vi "ADC Get Capabilities.vi"(7 "Initialize HW? (False)":bool, 8 "error in":errorcluster, 10 "parameters":T1, 11 "adc session in":T5={"niScope"={"channel cfg"=[], "sessions"=[], "multi cards"=FALSE, "channels"=0, "type"=enum."n/a", "memory [B/chn]"=0, "ext. clock [Hz]"=0.0, "samples count"=0, "use streaming"=FALSE, "proc setup"={"packet size [smpl]"=0, "current timeout [s]"=0.0, "blk2blk timeout [s]"=0.0, "event time"=timestamp(0 s since 1904-01-01), "temp sampl T [s]"=0.0, "data queue"=refnum, "stop notifier"=refnum, "proc ref"=refnum}, "sample width [B]"=0, "ranges [V]"=[], "trigger setup"={"coupling"=1, "level [V]"=0.0, "slope"=0, "mode"=enum."Immediate", "pre-trigger [%]"=0.0}, "fs [Hz]"=0.0, "bitres [bit]"=0, "clock source"=enum."VAL_NO_SOURCE"}, "3458A"={"channels"=[], "sync unit"={"VISA"="", "type"=enum."Picotest U6200A"}, "awg unit"={"type"=enum."Agilent 331xxA to 332xxA", "VISA"="", "enable 10MHz ref"=FALSE, "cmi ckd2"={"VISA"="", "clock source"=enum."Auto", "manual ref clk"=FALSE, "ref clock [Hz]"=0.0, "div mode"=enum."Set divisor directly"}, "cmi sync v3"={"VISA"="", "baud rate [bd/s]"=115200, "source"=enum."Auto", "hv range"=enum."1kV", "fsrc is fixed"=FALSE, "fsrc [Hz]"=10000000.0, "freq integ [s]"=1.0, "freq filter"=5, "trig level"=enum."TTL 5V", "chn1 mode"=enum."Source divider", "chn1 level"=enum."Positive 5V", "chn2 mode"=enum."Source divider", "chn2 level"=enum."Positive 5V", "chn2 div"=1, "chn3 mode"=enum."Chn 1 Active", "chn3 level"=enum."Positive 5V", "chn1 div entry"=enum."Calculate nearest divisor from measured fx", "chn1 dev limit [%]"=1.0, "chn1 check dev"=FALSE}, "trigger"={"source"=enum."Immediate", "slope"=enum."POS", "coupling"=enum."DC", "level [V]"=0.0, "hysteresis [V]"=0.0, "pre-trigger [%]"=0.0}, "HMF2500 cfg"={"Baud Rate"=9600, "Parity"=0, "Data Bits"=8, "Flow Control"=4}}, "sync mode"=enum."MASTER-SLAVE, MASTER clocked by TIMER", "streaming mode"=FALSE, "idn mode"=enum."Auto", "sampling mode"=enum."DCV", "sample memory [B]"=0, "proc setup"={"channel id"=0, "packet size [smpl]"=0, "current timeout [s]"=0.0, "blk2blk timeout [s]"=0.0, "event time"=timestamp(0 s since 1904-01-01), "stop notifier"=refnum, "data queues"=[], "proc refs"=[], "bus semaphore"=refnum}, "sample size [B]"=0, "sample count"=0, "aux data"={"channel id"=0, "valid?"=[], "gain [V]"=[], "timestamp [s]"=[], "Ts [s]"=0.0, "abs timestamp"=timestamp(0 s since 1904-01-01), "t [deg C]"=[], "multiplex timestamp [s]"=-1.0, "only multiplex?"=FALSE, "multiplex smpl offset"=0, "overflow?"=FALSE}, "ranges [V]"=[], "aperture [s]"=0.0, "LEVEL trigger"={"edge"=enum."POS", "level [V]"=0.0, "coupling"=enum."DC"}, "trigger mode"=enum."AUTO", "measure temp.?"=FALSE, "disp mesages"=[], "shared bus?"=FALSE, "disable display?"=FALSE, "aper mode"=enum."Manual", "aper rules"=[], "multiplex"={"cycles"=0, "delay [s]"=0.0, "enabled"=FALSE, "overhead [s]"=1.0, "tot smpls"=0, "sub-rec"=0, "overhead [%]"=0.0, "emulated"=FALSE}, "F8588 lpf"=enum."Off", "F8588 pll"=enum."Off", "F8588 couple"=enum."DC, auto", "fs"={"freq mode"=enum."fs or Ts", "fs [Hz]"=0.0, "fref [Hz]"=0.0, "mul"=0.0, "div"=0.0}, "fs mode"=enum."fs or Ts"}, "dsdll"={"dsdll"={"dsdll path"=path "", "dsdll handle"=[], "output devices"=[], "capture devices"=[]}, "channels"=0, "device id"=0, "channel idns"=[], "proc setup"={"packet size [smpl]"=0, "current timeout [s]"=0.0, "blk2blk timeout [s]"=0.0, "event time"=timestamp(0 s since 1904-01-01), "data queue"=refnum, "stop notifier"=refnum, "proc ref"=refnum}, "samples count"=0, "fs [Hz]"=0.0}, "type"=enum."niScope", "channel idn str"=[], "aux instr idn str"=[], "modified?"=FALSE, "simadc"={"channels"=[], "range [V]"=0.0, "Ts step [s]"=0.0, "time [s]"=0.0, "fs [Hz]"=0.0, "count"=0, "smpl offset"=0, "set count"=0, "bit res"=0}, "force rst?"=FALSE, "exit mode"=enum."Immediate reset", "exit dly"=0.0, "exit tmr"=timestamp(0 s since 1904-01-01), "busy?"=FALSE, "accessed?"=FALSE, "multiplex"={"Type"=enum."Dummy", "gen com ssn"={"visa"="", "primary"=enum."None", "secondary"=enum."None", "channels"=[]}, "delay before [s]"=0.0, "delay post [s]"=0.0, "sequence"=[], "enabled"=FALSE, "ref timestamp [s]"=0.0, "idn string"="", "dev niScope"="", "niScope idx"=0, "QPMX ssn"={"visa"="", "switch mode"=enum."Switched by TWM", "sequence"=[], "timing delays"=[], "polarity"=enum."Positive", "ss delay (s)"=2.0, "internal timer (s)"=1.0, "Last loaded sequence file"=path "", "startup delay (s)"=2.0}, "VISA mux ssn"={"VISA"="", "paths"=[], "idn command"="", "serial cfg"={"Baud rate"=9600, "Data bits"=8, "Parity"=0, "Stop bits"=10, "Flow control"=0, "End Mode Read"=enum."None", "End Mode Write"=enum."None", "Term character"=0, "Term enable"=FALSE}}}, "keysight dso"={"VISA"="", "channels"=[], "bw limit [Hz]"=0.0, "resolution"=enum."Basic", "trig noise reject"=enum."Normal", "N"=0, "trigger config"={"trigger source"=enum."Immediate", "trigger slope"=enum."Negative", "level [V]"=0.0, "hysteresis [V]"=0.001, "pre-trig [%]"=50}, "fs [Hz]"=0.0, "timeout stop"=timestamp(0 s since 1904-01-01), "waiting for opc"=FALSE, "fetch offset [smpl]"=0, "abs timestamp"=timestamp(0 s since 1904-01-01), "ranges [V]"=[], "decimation"=1.0, "ext ref"=FALSE, "emulate aperture"=FALSE, "model"=enum."DSO91304"}, "cdaq"={"mclk [Hz]"=12800000.0, "ADC task"="", "mclk reference"="", "fs [Hz]"=50000.0, "queue adc cmd"=refnum, "queue adc data"=refnum, "adc proc ref"=refnum, "channels"=[], "last channels"=[], "timeout"=timestamp(0 s since 1904-01-01), "N"=1000, "mclk mode"=enum."Free running", "ext mclk source"=""}, "ignore overload"=FALSE, "ADS127L21"={"VISA"="", "chn list"=[], "record size"=0, "phys. channels"=0, "adc fifo size"=0, "channels"=[], "ext refclk?"=FALSE, "fs [Hz]"=0.0, "ext refclk [Hz]"=0.0, "meas refclk [Hz]"=0.0, "EXTOUT mode"=enum."ADCCLK", "EXTOUT polarity"=enum."NORM", "EXTOUT divisor"=0}} {"ADS127L21"."channels"."Channel" min=1 max=8 step=1; "cdaq"."last channels"."Channel id" min=0 step=1; "cdaq"."channels"."Channel id" min=0 step=1; "keysight dso"."decimation" min=1.0; "keysight dso"."bw limit [Hz]" format="%#_6p"; "keysight dso"."channels"."Offset [V]" format="%#_6p"; "keysight dso"."channels"."Range [Vpk]" min=0.0 format="%#_6p"; "keysight dso"."channels"."Channel" min=1; "multiplex"."VISA mux ssn"."serial cfg"."Flow control" items=["None", "XON/XOFF", "CTS/RTS", "XON/XOFF + CTS/RTS", "DTR/DSR", "XON/XOFF + DTR/DSR"]; "multiplex"."VISA mux ssn"."serial cfg"."Stop bits" items=["1 bit"=10, "1.5 bits"=15, "2 bits"=20]; "multiplex"."VISA mux ssn"."serial cfg"."Parity" items=["None", "Odd", "Even", "Mark", "Space"]; "multiplex"."VISA mux ssn"."serial cfg"."Data bits" items=["5 bits"=5, "6 bits"=6, "7 bits"=7, "8 bits"=8]; "multiplex"."VISA mux ssn"."serial cfg"."Baud rate" items=["150 Bd"=150, "300 Bd"=300, "600 Bd"=600, "1200 Bd"=1200, "2400 Bd"=2400, "4800 Bd"=4800, "9600 Bd"=9600, "19.2 kBd"=19200, "38.4 kBd"=38400, "57.6 kBd"=57600, "115.2 kBd"=115200]; "multiplex"."QPMX ssn"."startup delay (s)" min=0.0 step=1.0; "multiplex"."QPMX ssn"."internal timer (s)" min=0.0 step=1.0; "multiplex"."QPMX ssn"."ss delay (s)" min=0.0 step=1.0; "multiplex"."QPMX ssn"."timing delays" min=1 max=255 step=1; "3458A"."awg unit"."HMF2500 cfg"."Flow Control" items=["None", "XON/XOFF", "RTS/CTS", "XON/XOFF & RTS/CTS", "DTR/DSR", "XON/XOFF & DTR/DSR"]; "3458A"."awg unit"."HMF2500 cfg"."Data Bits" items=["7"=7, "8"=8]; "3458A"."awg unit"."HMF2500 cfg"."Parity" items=["None", "Odd", "Even", "Mark", "Space"]; "3458A"."awg unit"."HMF2500 cfg"."Baud Rate" items=["300"=300, "600"=600, "1200"=1200, "2400"=2400, "4800"=4800, "9600"=9600, "19200"=19200]; "3458A"."awg unit"."cmi sync v3"."chn2 div" min=1 max=100000000 step=1; "3458A"."awg unit"."cmi sync v3"."fsrc [Hz]" format="%_8p"; "3458A"."channels"."Range [Vpk]" min=0.0; "niScope"."trigger setup"."pre-trigger [%]" format="%.2f"; "niScope"."trigger setup"."level [V]" format="%.2f"; "niScope"."trigger setup"."coupling" items=["AC"=0, "DC"=1, "HF Reject"=3, "LF Reject"=4, "AC Plus HF Reject"=1001]; "niScope"."channel cfg"."Range [Vpk]" min=0.0; "niScope"."channel cfg"."Channel" min=0}) -> (0 "error out":errorcluster, 2 "capabilities":T2, 3 "adc session out":T5={"niScope"={"channel cfg"=[], "sessions"=[], "multi cards"=FALSE, "channels"=0, "type"=enum."n/a", "memory [B/chn]"=0, "ext. clock [Hz]"=0.0, "samples count"=0, "use streaming"=FALSE, "proc setup"={"packet size [smpl]"=0, "current timeout [s]"=0.0, "blk2blk timeout [s]"=0.0, "event time"=timestamp(0 s since 1904-01-01), "temp sampl T [s]"=0.0, "data queue"=refnum, "stop notifier"=refnum, "proc ref"=refnum}, "sample width [B]"=0, "ranges [V]"=[], "trigger setup"={"coupling"=1, "level [V]"=0.0, "slope"=0, "mode"=enum."Immediate", "pre-trigger [%]"=0.0}, "fs [Hz]"=0.0, "bitres [bit]"=0, "clock source"=enum."VAL_NO_SOURCE"}, "3458A"={"channels"=[], "sync unit"={"VISA"="", "type"=enum."Picotest U6200A"}, "awg unit"={"type"=enum."Agilent 331xxA to 332xxA", "VISA"="", "enable 10MHz ref"=FALSE, "cmi ckd2"={"VISA"="", "clock source"=enum."Auto", "manual ref clk"=FALSE, "ref clock [Hz]"=0.0, "div mode"=enum."Set divisor directly"}, "cmi sync v3"={"VISA"="", "baud rate [bd/s]"=115200, "source"=enum."Auto", "hv range"=enum."1kV", "fsrc is fixed"=FALSE, "fsrc [Hz]"=10000000.0, "freq integ [s]"=1.0, "freq filter"=5, "trig level"=enum."TTL 5V", "chn1 mode"=enum."Source divider", "chn1 level"=enum."Positive 5V", "chn2 mode"=enum."Source divider", "chn2 level"=enum."Positive 5V", "chn2 div"=1, "chn3 mode"=enum."Chn 1 Active", "chn3 level"=enum."Positive 5V", "chn1 div entry"=enum."Calculate nearest divisor from measured fx", "chn1 dev limit [%]"=1.0, "chn1 check dev"=FALSE}, "trigger"={"source"=enum."Immediate", "slope"=enum."POS", "coupling"=enum."DC", "level [V]"=0.0, "hysteresis [V]"=0.0, "pre-trigger [%]"=0.0}, "HMF2500 cfg"={"Baud Rate"=9600, "Parity"=0, "Data Bits"=8, "Flow Control"=4}}, "sync mode"=enum."MASTER-SLAVE, MASTER clocked by TIMER", "streaming mode"=FALSE, "idn mode"=enum."Auto", "sampling mode"=enum."DCV", "sample memory [B]"=0, "proc setup"={"channel id"=0, "packet size [smpl]"=0, "current timeout [s]"=0.0, "blk2blk timeout [s]"=0.0, "event time"=timestamp(0 s since 1904-01-01), "stop notifier"=refnum, "data queues"=[], "proc refs"=[], "bus semaphore"=refnum}, "sample size [B]"=0, "sample count"=0, "aux data"={"channel id"=0, "valid?"=[], "gain [V]"=[], "timestamp [s]"=[], "Ts [s]"=0.0, "abs timestamp"=timestamp(0 s since 1904-01-01), "t [deg C]"=[], "multiplex timestamp [s]"=-1.0, "only multiplex?"=FALSE, "multiplex smpl offset"=0, "overflow?"=FALSE}, "ranges [V]"=[], "aperture [s]"=0.0, "LEVEL trigger"={"edge"=enum."POS", "level [V]"=0.0, "coupling"=enum."DC"}, "trigger mode"=enum."AUTO", "measure temp.?"=FALSE, "disp mesages"=[], "shared bus?"=FALSE, "disable display?"=FALSE, "aper mode"=enum."Manual", "aper rules"=[], "multiplex"={"cycles"=0, "delay [s]"=0.0, "enabled"=FALSE, "overhead [s]"=1.0, "tot smpls"=0, "sub-rec"=0, "overhead [%]"=0.0, "emulated"=FALSE}, "F8588 lpf"=enum."Off", "F8588 pll"=enum."Off", "F8588 couple"=enum."DC, auto", "fs"={"freq mode"=enum."fs or Ts", "fs [Hz]"=0.0, "fref [Hz]"=0.0, "mul"=0.0, "div"=0.0}, "fs mode"=enum."fs or Ts"}, "dsdll"={"dsdll"={"dsdll path"=path "", "dsdll handle"=[], "output devices"=[], "capture devices"=[]}, "channels"=0, "device id"=0, "channel idns"=[], "proc setup"={"packet size [smpl]"=0, "current timeout [s]"=0.0, "blk2blk timeout [s]"=0.0, "event time"=timestamp(0 s since 1904-01-01), "data queue"=refnum, "stop notifier"=refnum, "proc ref"=refnum}, "samples count"=0, "fs [Hz]"=0.0}, "type"=enum."niScope", "channel idn str"=[], "aux instr idn str"=[], "modified?"=FALSE, "simadc"={"channels"=[], "range [V]"=0.0, "Ts step [s]"=0.0, "time [s]"=0.0, "fs [Hz]"=0.0, "count"=0, "smpl offset"=0, "set count"=0, "bit res"=0}, "force rst?"=FALSE, "exit mode"=enum."Immediate reset", "exit dly"=0.0, "exit tmr"=timestamp(0 s since 1904-01-01), "busy?"=FALSE, "accessed?"=FALSE, "multiplex"={"Type"=enum."Dummy", "gen com ssn"={"visa"="", "primary"=enum."None", "secondary"=enum."None", "channels"=[]}, "delay before [s]"=0.0, "delay post [s]"=0.0, "sequence"=[], "enabled"=FALSE, "ref timestamp [s]"=0.0, "idn string"="", "dev niScope"="", "niScope idx"=0, "QPMX ssn"={"visa"="", "switch mode"=enum."Switched by TWM", "sequence"=[], "timing delays"=[], "polarity"=enum."Positive", "ss delay (s)"=2.0, "internal timer (s)"=1.0, "Last loaded sequence file"=path "", "startup delay (s)"=2.0}, "VISA mux ssn"={"VISA"="", "paths"=[], "idn command"="", "serial cfg"={"Baud rate"=9600, "Data bits"=8, "Parity"=0, "Stop bits"=10, "Flow control"=0, "End Mode Read"=enum."None", "End Mode Write"=enum."None", "Term character"=0, "Term enable"=FALSE}}}, "keysight dso"={"VISA"="", "channels"=[], "bw limit [Hz]"=0.0, "resolution"=enum."Basic", "trig noise reject"=enum."Normal", "N"=0, "trigger config"={"trigger source"=enum."Immediate", "trigger slope"=enum."Negative", "level [V]"=0.0, "hysteresis [V]"=0.001, "pre-trig [%]"=50}, "fs [Hz]"=0.0, "timeout stop"=timestamp(0 s since 1904-01-01), "waiting for opc"=FALSE, "fetch offset [smpl]"=0, "abs timestamp"=timestamp(0 s since 1904-01-01), "ranges [V]"=[], "decimation"=1.0, "ext ref"=FALSE, "emulate aperture"=FALSE, "model"=enum."DSO91304"}, "cdaq"={"mclk [Hz]"=12800000.0, "ADC task"="", "mclk reference"="", "fs [Hz]"=50000.0, "queue adc cmd"=refnum, "queue adc data"=refnum, "adc proc ref"=refnum, "channels"=[], "last channels"=[], "timeout"=timestamp(0 s since 1904-01-01), "N"=1000, "mclk mode"=enum."Free running", "ext mclk source"=""}, "ignore overload"=FALSE, "ADS127L21"={"VISA"="", "chn list"=[], "record size"=0, "phys. channels"=0, "adc fifo size"=0, "channels"=[], "ext refclk?"=FALSE, "fs [Hz]"=0.0, "ext refclk [Hz]"=0.0, "meas refclk [Hz]"=0.0, "EXTOUT mode"=enum."ADCCLK", "EXTOUT polarity"=enum."NORM", "EXTOUT divisor"=0}} {"ADS127L21"."channels"."Channel" min=1 max=8 step=1; "cdaq"."last channels"."Channel id" min=0 step=1; "cdaq"."channels"."Channel id" min=0 step=1; "keysight dso"."decimation" min=1.0; "keysight dso"."bw limit [Hz]" format="%#_6p"; "keysight dso"."channels"."Offset [V]" format="%#_6p"; "keysight dso"."channels"."Range [Vpk]" min=0.0 format="%#_6p"; "keysight dso"."channels"."Channel" min=1; "multiplex"."VISA mux ssn"."serial cfg"."Flow control" items=["None", "XON/XOFF", "CTS/RTS", "XON/XOFF + CTS/RTS", "DTR/DSR", "XON/XOFF + DTR/DSR"]; "multiplex"."VISA mux ssn"."serial cfg"."Stop bits" items=["1 bit"=10, "1.5 bits"=15, "2 bits"=20]; "multiplex"."VISA mux ssn"."serial cfg"."Parity" items=["None", "Odd", "Even", "Mark", "Space"]; "multiplex"."VISA mux ssn"."serial cfg"."Data bits" items=["5 bits"=5, "6 bits"=6, "7 bits"=7, "8 bits"=8]; "multiplex"."VISA mux ssn"."serial cfg"."Baud rate" items=["150 Bd"=150, "300 Bd"=300, "600 Bd"=600, "1200 Bd"=1200, "2400 Bd"=2400, "4800 Bd"=4800, "9600 Bd"=9600, "19.2 kBd"=19200, "38.4 kBd"=38400, "57.6 kBd"=57600, "115.2 kBd"=115200]; "multiplex"."QPMX ssn"."startup delay (s)" min=0.0 step=1.0; "multiplex"."QPMX ssn"."internal timer (s)" min=0.0 step=1.0; "multiplex"."QPMX ssn"."ss delay (s)" min=0.0 step=1.0; "multiplex"."QPMX ssn"."timing delays" min=1 max=255 step=1; "3458A"."awg unit"."HMF2500 cfg"."Flow Control" items=["None", "XON/XOFF", "RTS/CTS", "XON/XOFF & RTS/CTS", "DTR/DSR", "XON/XOFF & DTR/DSR"]; "3458A"."awg unit"."HMF2500 cfg"."Data Bits" items=["7"=7, "8"=8]; "3458A"."awg unit"."HMF2500 cfg"."Parity" items=["None", "Odd", "Even", "Mark", "Space"]; "3458A"."awg unit"."HMF2500 cfg"."Baud Rate" items=["300"=300, "600"=600, "1200"=1200, "2400"=2400, "4800"=4800, "9600"=9600, "19200"=19200]; "3458A"."awg unit"."cmi sync v3"."chn2 div" min=1 max=100000000 step=1; "3458A"."awg unit"."cmi sync v3"."fsrc [Hz]" format="%_8p"; "3458A"."channels"."Range [Vpk]" min=0.0; "niScope"."trigger setup"."pre-trigger [%]" format="%.2f"; "niScope"."trigger setup"."level [V]" format="%.2f"; "niScope"."trigger setup"."coupling" items=["AC"=0, "DC"=1, "HF Reject"=3, "LF Reject"=4, "AC Plus HF Reject"=1001]; "niScope"."channel cfg"."Range [Vpk]" min=0.0; "niScope"."channel cfg"."Channel" min=0})   [LabVIEW 2020]
doc: "This VI returns cluster of capabilities for selected HW. Note that to make it work the session must be either live (opened) or at least were opened and closed so the HW paramter data are in the session. Alternatively use option 'initialize HW'. That will open and close the HW so the data are read. Keep in mind this option may take some time so it should not be done every second in the GUI but for instance just once when GUI panel opens. Note that some of the paramters may not be valid if the input parameters are not assigned."
uses:
  drivers/DMM/3458A Virtual Digitizer.lvlib
  ADC Capabilities.ctl
  ADC Sampling Rate Step Mode.ctl
  drivers/niScope/niScope Virtual Digitizer.lvlib
  drivers/AWG/AWG Clock Setup Mode.ctl
  drivers/AWG/AWG.lvlib
  drivers/niScope/niScope Virtual Channel Mode.ctl
  drivers/niScope/niScope Virtual Channel Input Z.ctl
  drivers/niScope/niScope Virtual Channel Coupling.ctl
  drivers/niScope/niScope Virtual Channel Config.ctl
  drivers/niScope/niScope Type.ctl
  drivers/niScope/niScope Data Packet.ctl
  drivers/niScope/niScope Digitizing Process Options.ctl
  drivers/niScope/niScope Session.ctl
  drivers/DMM/3458A Virtual Channel Config.ctl
  drivers/Counter/Counter Type.ctl
  drivers/Counter/Counter.lvlib
  drivers/Counter/Counter Session.ctl
  drivers/AWG/AWG Type.ctl
  drivers/AWG/AWG Session.ctl
  drivers/DMM/3458A Sync Mode.ctl
  drivers/DMM/3458A Idn Mode.ctl
  drivers/DMM/3458A Digitizing Low Levels/Configure/Sampling Mode.ctl
  drivers/DMM/3458A Digitizing Low Levels/3458A Digitizing Low Levels.lvlib
  drivers/DMM/3458A Data Packet.ctl
  drivers/DMM/3458A Digitizing Process Options.ctl
  drivers/DMM/3458A Aux Record Data.ctl
  drivers/DMM/3458A Digitizer Session.ctl
  ADC Type.ctl
  ADC Session.ctl
  ADC Capabilities Parameters.ctl
  drivers/dsdll/DSDLL Data Packet.ctl
  drivers/dsdll/DSDLL Virtual Digitizer.lvlib
  drivers/dsdll/DSDLL Process Config.ctl
  drivers/dsdll/DSDLL Session.ctl
  <instrlib>/niScope/Controls/niScope trigger coupling.ctl
  <instrlib>/niScope/Controls/niScope trigger slope.ctl
  drivers/niScope/niScope Trigger Setup.ctl
  drivers/DMM/3458A Digitizing Low Levels/Configure/Level Setup.ctl
  drivers/DMM/3458A Digitizing Low Levels/Configure/First Sample Trigger.ctl
  drivers/simulated_adc/SimAdc Channel Cfg.ctl
  drivers/simulated_adc/SimAdc Config.ctl
  drivers/niScope/niScope Reference Clock.ctl
  drivers/DMM/3458A Aperture Selection Mode.ctl
  drivers/DMM/3458A Multiplexing Config.ctl
  ADC On Close Action.ctl
  Multiplexer/MPX Type.ctl
  drivers/Multiplexers/Generic COM/GCOMM Signal.ctl
  drivers/Multiplexers/Generic COM/GCOMM Logic State.ctl
  drivers/Multiplexers/Generic COM/GCOMM Virtual Channel.ctl
  drivers/Multiplexers/Generic COM/GCOMM Session.ctl
  Multiplexer/MPX Session.ctl
  drivers/Agilent DSO 90000/Virtual Digitizer/KeDSO Virtual Channel.ctl
  drivers/Agilent DSO 90000/Virtual Digitizer/KeDSO Trigger Source.ctl
  drivers/Agilent DSO 90000/Virtual Digitizer/KeDSO Trigger Setup.ctl
  drivers/Agilent DSO 90000/Virtual Digitizer/KeDSO session.ctl
  drivers/cdaq/low_level_old/cdaq_anal_adc_command.ctl
  drivers/cdaq/low_level_old/cdaq_anal_adc_data.ctl
  drivers/cdaq/cDAQ Virtual Channel.ctl
  drivers/cdaq/cDAQ Session.ctl
  drivers/Fluke 8588A/F8588A Low Pass Filter.ctl
  drivers/Fluke 8588A/F8588A Phase Lock.ctl
  drivers/Fluke 8588A/F8588A Coupling.ctl
  drivers/AWG/CMI Clock Divider v2/CMI ckd2 Source Mode.ctl
  drivers/AWG/CMI Clock Divider v2/CMI ckd2 Session.ctl
  drivers/dsdll/dsdll/dsdll_device_record.ctl
  drivers/dsdll/dsdll/dsdll.lvlib
  drivers/dsdll/dsdll/dsdll_instance.ctl
  drivers/cdaq/cDAQ Master Clock Mode.ctl
  drivers/Multiplexers/QPMX/QPMX switch mode.ctl
  drivers/Multiplexers/QPMX/QPMX polarity.ctl
  drivers/Multiplexers/Generic COM/QPMX Session.ctl
  drivers/AWG/CMI Sync V3/Configure/CMI Sync V3 Reference Clock Source.ctl
  drivers/AWG/CMI Sync V3/CMI Sync Unit V3.lvlib
  drivers/AWG/CMI Sync V3/Configure/CMI Sync V3 HV input Range.ctl
  drivers/AWG/CMI Sync V3/Configure/CMI Sync V3 Trigger Input Level.ctl
  drivers/AWG/CMI Sync V3/Configure/CMI Sync V3 Channel 1 Mode.ctl
  drivers/AWG/CMI Sync V3/Configure/CMI Sync V3 Channel Output Levels.ctl
  drivers/AWG/CMI Sync V3/Configure/CMI Sync V3 Channel 2 Mode.ctl
  drivers/AWG/CMI Sync V3/Configure/CMI Sync V3 Channel 3 Mode.ctl
  drivers/AWG/CMI Sync V3/CMI Sync V3 session.ctl
  drivers/AWG/CMI Clock Divider v2/CMI ckd2 Divisor Mode.ctl
  drivers/AWG/CMI Sync V3/Configure/CMI Sync V3 Channel 1 Divisor Entry Mode.ctl
  ADC Trig Mode Source.ctl
  ADC Trig Coupling.ctl
  ADC Trig Slope.ctl
  ADC Trig Config.ctl
  drivers/AWG/RaS HMF2500/HMF2500 Config.ctl
  drivers/DMM/3458A Sampling Rate.ctl
  drivers/Multiplexers/Generic VISA commands/GVISA Mux Path Entry.ctl
  drivers/Multiplexers/Generic VISA commands/met_serial_setup.ctl
  drivers/Multiplexers/Generic VISA commands/GVISA Mux Session.ctl
  drivers/DMM/3458A Sample Rate Mode.ctl
  drivers/Agilent DSO 90000/Virtual Digitizer/KeDSO High Resolution Mode.ctl
  drivers/Agilent DSO 90000/Public/Utility/DSO type.ctl
  drivers/Agilent DSO 90000/Agilent 90000 Series.lvlib
  drivers/CMI_ADS127L21/CMI ADS127L21 - Input Range.ctl
  drivers/CMI_ADS127L21/CMI ADS127L21 - Input Mode.ctl
  drivers/CMI_ADS127L21/CMI ADS127L21 - Input Impedance.ctl
  drivers/CMI_ADS127L21/CMI ADS127L21 - Record Channel.ctl
  drivers/CMI_ADS127L21/CMI ADS127L21 - EXTOUT Mode.ctl
  drivers/CMI_ADS127L21/CMI ADS127L21 - EXTOUT Polarity.ctl
  drivers/CMI_ADS127L21/CMI ADS127L21 - Session.ctl
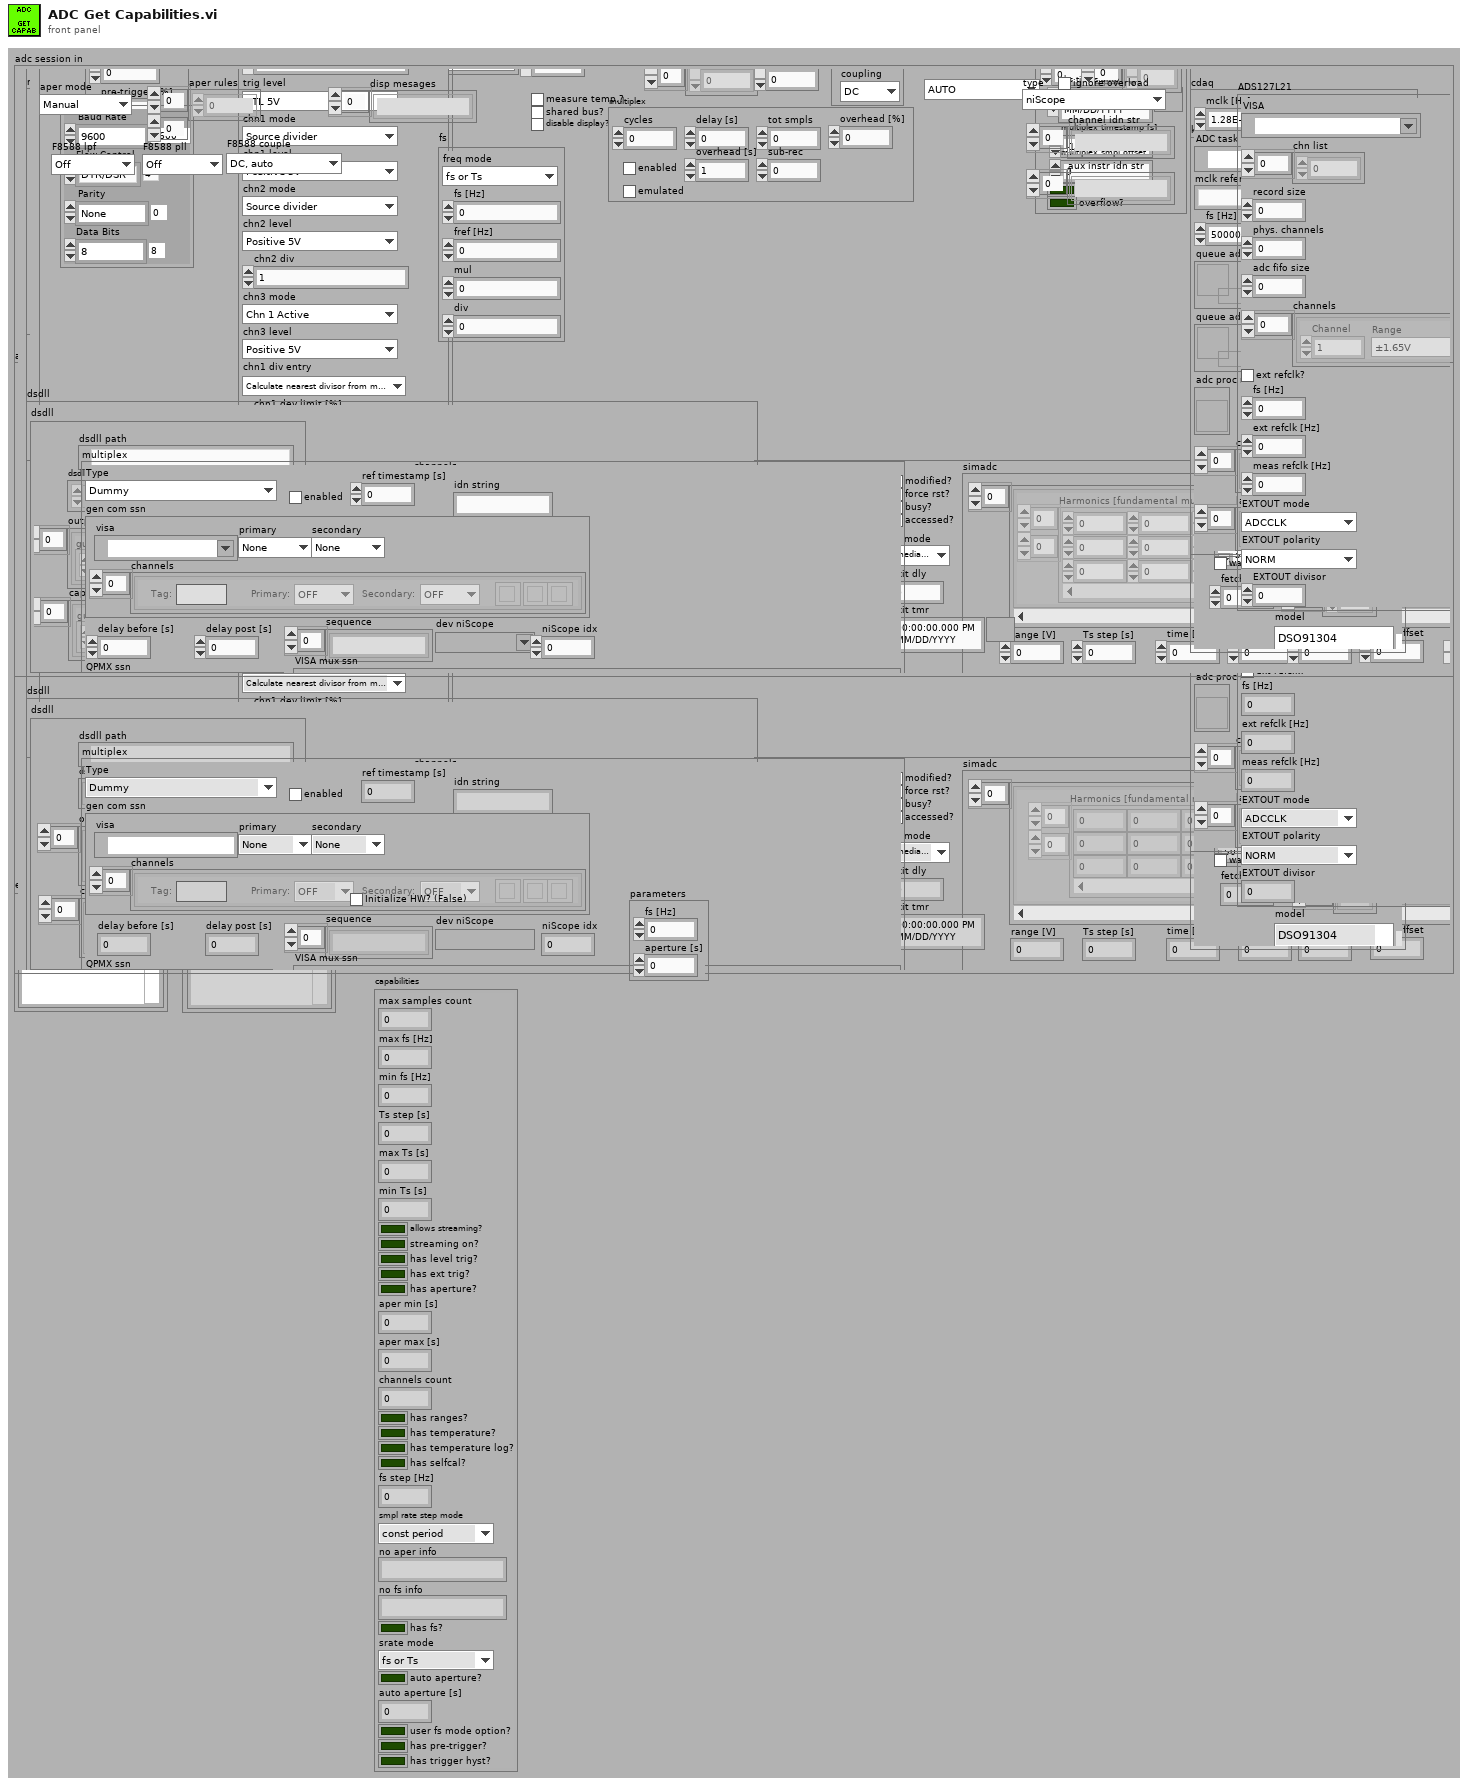
[diagram p1: front panel]
types:
  T1 = typedef "ADC Capabilities Parameters.ctl" = cluster{"fs [Hz]":dbl, "aperture [s]":dbl}
  T2 = typedef "ADC Capabilities.ctl" = cluster{"max samples count":i64, "max fs [Hz]":ext, "min fs [Hz]":ext, "Ts step [s]":ext, "max Ts [s]":ext, "min Ts [s]":ext, "allows streaming?":bool, "streaming on?":bool, "has level trig?":bool, "has ext trig?":bool, "has aperture?":bool, "aper min [s]":dbl, "aper max [s]":dbl, "channels count":i32, "has ranges?":bool, "has temperature?":bool, "has temperature log?":bool, "has selfcal?":bool, "fs step [Hz]":ext, "smpl rate step mode":T3, "no aper info":string, "no fs info":string, "has fs?":bool, "srate mode":T4, "auto aperture?":bool, "auto aperture [s]":ext, "user fs mode option?":bool, "has pre-trigger?":bool, "has trigger hyst?":bool}
  T3 = typedef "ADC Sampling Rate Step Mode.ctl" = enum16{"const period", "const frequency"}
  T4 = typedef "AWG.lvlib/AWG Clock Setup Mode.ctl" = enum16{"fs or Ts", "fs or Ts with fref", "fref/N", "fref*M/N", "fref*Ratio"}
  T5 = typedef "ADC Session.ctl" = cluster{"niScope":T6, "3458A":T17, "dsdll":T55, "type":T59, "channel idn str":string[], "aux instr idn str":string[], "modified?":bool, "simadc":T60, "force rst?":bool, "exit mode":T62, "exit dly":dbl, "exit tmr":timestamp, "busy?":bool, "accessed?":bool, "multiplex":T63, "keysight dso":T75, "cdaq":T81, "ignore overload":bool, "ADS127L21":T84}
  T6 = typedef "niScope Virtual Digitizer.lvlib/niScope Session.ctl" = cluster{"channel cfg":T7[], "sessions":refnum<k20>[], "multi cards":bool, "channels":i32, "type":T11, "memory [B/chn]":i32, "ext. clock [Hz]":dbl, "samples count":i64, "use streaming":bool, "proc setup":T12, "sample width [B]":i32, "ranges [V]":dbl[], "trigger setup":T13, "fs [Hz]":dbl, "bitres [bit]":i32, "clock source":T16}
  T7 = typedef "niScope Virtual Digitizer.lvlib/niScope Virtual Channel Config.ctl" = cluster{"Address":refnum<k15>, "Channel":i32, "Mode":T8, "Input Z":T9, "Coupling":T10, "Range [Vpk]":dbl, "btn clr":bool, "btn up":bool, "btn down":bool}
  T8 = typedef "niScope Virtual Digitizer.lvlib/niScope Virtual Channel Mode.ctl" = enum16{"Single ended", "Unbal. differential", "Differential"}
  T9 = typedef "niScope Virtual Digitizer.lvlib/niScope Virtual Channel Input Z.ctl" = enum16{"1 MOhm", "50 Ohm"}
  T10 = typedef "niScope Virtual Digitizer.lvlib/niScope Virtual Channel Coupling.ctl" = enum16{"AC", "DC", "GND"}
  T11 = typedef "niScope Virtual Digitizer.lvlib/niScope Type.ctl" = enum16{"n/a", "5922"}
  T12 = typedef "niScope Virtual Digitizer.lvlib/niScope Digitizing Process Options.ctl" = cluster{"packet size [smpl]":i64, "current timeout [s]":dbl, "blk2blk timeout [s]":dbl, "event time":timestamp, "temp sampl T [s]":dbl, "data queue":refnum<queue>, "stop notifier":refnum<notifier>, "proc ref":refnum<vi>}
  T13 = typedef "niScope Virtual Digitizer.lvlib/niScope Trigger Setup.ctl" = cluster{"coupling":T14, "level [V]":dbl, "slope":T15, "mode":enum16{"Immediate", "External", "Level"}, "pre-trigger [%]":dbl}
  T14 = typedef "niScope trigger coupling.ctl" = u16
  T15 = typedef "niScope trigger slope.ctl" = i32
  T16 = typedef "niScope Virtual Digitizer.lvlib/niScope Reference Clock.ctl" = enum16{"VAL_NO_SOURCE", "VAL_CLK_IN", "VAL_PXI_CLOCK", "VAL_EXTERNAL"}
  T17 = typedef "3458A Virtual Digitizer.lvlib/3458A Digitizer Session.ctl" = cluster{"channels":T18[], "sync unit":T19, "awg unit":T21, "sync mode":T40, "streaming mode":bool, "idn mode":T41, "sampling mode":T42, "sample memory [B]":i32, "proc setup":T43, "sample size [B]":i32, "sample count":i32, "aux data":T45, "ranges [V]":dbl[], "aperture [s]":dbl, "LEVEL trigger":T46, "trigger mode":T47, "measure temp.?":bool, "disp mesages":string[], "shared bus?":bool, "disable display?":bool, "aper mode":T48, "aper rules":dbl[][], "multiplex":T49, "F8588 lpf":T50, "F8588 pll":T51, "F8588 couple":T52, "fs":T53, "fs mode":T54}
  T18 = typedef "3458A Virtual Digitizer.lvlib/3458A Virtual Channel Config.ctl" = cluster{"VISA":refnum<visa-resource-name>, "Range [Vpk]":dbl, "btn clr":bool, "btn up":bool, "btn down":bool, "F8588":bool, "F8588 guard":bool}
  T19 = typedef "Counter.lvlib/Counter Session.ctl" = cluster{"VISA":refnum<visa-resource-name>, "type":T20}
  T20 = typedef "Counter.lvlib/Counter Type.ctl" = enum16{"Picotest U6200A", "dummy"}
  T21 = typedef "AWG.lvlib/AWG Session.ctl" = cluster{"type":T22, "VISA":refnum<visa-resource-name>, "enable 10MHz ref":bool, "cmi ckd2":T23, "cmi sync v3":T26, "trigger":T35, "HMF2500 cfg":T39}
  T22 = typedef "AWG.lvlib/AWG Type.ctl" = enum16{"Agilent 331xxA to 332xxA", "Agilent 335xxA to 336xxA", "Tektronix AFG3101C", "R&S HMF25xx", "CMI Clock Divider v2", "CMI Sync Unit V3", "dummy"}
  T23 = typedef "AWG.lvlib/CMI ckd2 Session.ctl" = cluster{"VISA":refnum<visa-resource-name>, "clock source":T24, "manual ref clk":bool, "ref clock [Hz]":dbl, "div mode":T25}
  T24 = typedef "AWG.lvlib/CMI ckd2 Source Mode.ctl" = enum16{"Auto", "LF clock", "HF clock", "Internal"}
  T25 = typedef "AWG.lvlib/CMI ckd2 Divisor Mode.ctl" = enum16{"Set divisor directly", "Set divisor by frequency"}
  T26 = typedef "AWG.lvlib/CMI Sync Unit V3.lvlib/CMI Sync V3 session.ctl" = cluster{"VISA":refnum<visa-resource-name>, "baud rate [bd/s]":i32, "source":T27, "hv range":T28, "fsrc is fixed":bool, "fsrc [Hz]":dbl, "freq integ [s]":dbl, "freq filter":i32, "trig level":T29, "chn1 mode":T30, "chn1 level":T31, "chn2 mode":T32, "chn2 level":T31, "chn2 div":i32, "chn3 mode":T33, "chn3 level":T31, "chn1 div entry":T34, "chn1 dev limit [%]":dbl, "chn1 check dev":bool}
  T27 = typedef "AWG.lvlib/CMI Sync Unit V3.lvlib/CMI Sync V3 Reference Clock Source.ctl" = enum16{"Auto", "Internal", "Logic", "Sine", "HV"}
  T28 = typedef "AWG.lvlib/CMI Sync Unit V3.lvlib/CMI Sync V3 HV input Range.ctl" = enum16{"10V", "60V", "250V", "1kV"}
  T29 = typedef "AWG.lvlib/CMI Sync Unit V3.lvlib/CMI Sync V3 Trigger Input Level.ctl" = enum16{"LVCMOS 3V3", "TTL 5V"}
  T30 = typedef "AWG.lvlib/CMI Sync Unit V3.lvlib/CMI Sync V3 Channel 1 Mode.ctl" = enum16{"Source divider", "DDS absolute", "DDS ratio", "DDS ratio M/N"}
  T31 = typedef "AWG.lvlib/CMI Sync Unit V3.lvlib/CMI Sync V3 Channel Output Levels.ctl" = enum16{"Positive 3V3", "Negative 3V3", "Positive 5V", "Negative 5V"}
  T32 = typedef "AWG.lvlib/CMI Sync Unit V3.lvlib/CMI Sync V3 Channel 2 Mode.ctl" = enum16{"Source divider", "Chn 1 divide"}
  T33 = typedef "AWG.lvlib/CMI Sync Unit V3.lvlib/CMI Sync V3 Channel 3 Mode.ctl" = enum16{"Chn 1 Active", "Chn 2 Active", "Chn 1 Trigger", "Chn 2 Trigger", "Gate", "PPS", "10MHz"}
  T34 = typedef "AWG.lvlib/CMI Sync Unit V3.lvlib/CMI Sync V3 Channel 1 Divisor Entry Mode.ctl" = enum16{"Set divisor directly", "Calculate nearest divisor from measured fx"}
  T35 = typedef "ADC Trig Config.ctl" = cluster{"source":T36, "slope":T37, "coupling":T38, "level [V]":dbl, "hysteresis [V]":dbl, "pre-trigger [%]":dbl}
  T36 = typedef "ADC Trig Mode Source.ctl" = enum16{"Immediate", "External", "Level"}
  T37 = typedef "ADC Trig Slope.ctl" = enum16{"POS", "NEG"}
  T38 = typedef "ADC Trig Coupling.ctl" = enum16{"DC", "AC"}
  T39 = typedef "AWG.lvlib/HMF2500 Config.ctl" = cluster{"Baud Rate":u32, "Parity":u16, "Data Bits":u16, "Flow Control":u16}
  T40 = typedef "3458A Virtual Digitizer.lvlib/3458A Sync Mode.ctl" = enum16{"MASTER-SLAVE, MASTER clocked by TIMER", "MASTER-SLAVE, MASTER clocked by AWG", "ALL clocked by AWG", "MASTER-SLAVE, ALL clocked by TIMER", "ALL clocked by AWG with DFLL"}
  T41 = typedef "3458A Virtual Digitizer.lvlib/3458A Idn Mode.ctl" = enum16{"Auto", "Sequential (chn A, chn B, ...)", "From calibration string"}
  T42 = typedef "3458A Virtual Digitizer.lvlib/3458A Digitizing Low Levels.lvlib/Sampling Mode.ctl" = enum16{"DCV", "DSDC", "DSAC"}
  T43 = typedef "3458A Virtual Digitizer.lvlib/3458A Digitizing Process Options.ctl" = cluster{"channel id":i32, "packet size [smpl]":i32, "current timeout [s]":dbl, "blk2blk timeout [s]":dbl, "event time":timestamp, "stop notifier":refnum<notifier>, "data queues":refnum<queue>[], "proc refs":refnum<vi>[], "bus semaphore":T44}
  T44 = typedef "Semaphore RefNum" = refnum<k1>
  T45 = typedef "3458A Virtual Digitizer.lvlib/3458A Aux Record Data.ctl" = cluster{"channel id":i32, "valid?":bool[], "gain [V]":dbl[], "timestamp [s]":dbl[], "Ts [s]":dbl, "abs timestamp":timestamp, "t [deg C]":dbl[], "multiplex timestamp [s]":dbl, "only multiplex?":bool, "multiplex smpl offset":i64, "overflow?":bool}
  T46 = typedef "3458A Virtual Digitizer.lvlib/3458A Digitizing Low Levels.lvlib/Level Setup.ctl" = cluster{"edge":enum16{"POS", "NEG"}, "level [V]":dbl, "coupling":enum16{"DC", "AC"}}
  T47 = typedef "3458A Virtual Digitizer.lvlib/3458A Digitizing Low Levels.lvlib/First Sample Trigger.ctl" = enum16{"AUTO", "EXT", "SYN", "SGL", "HOLD", "LEVEL"}
  T48 = typedef "3458A Virtual Digitizer.lvlib/3458A Aperture Selection Mode.ctl" = enum16{"Manual", "Maximum", "Table"}
  T49 = typedef "3458A Virtual Digitizer.lvlib/3458A Multiplexing Config.ctl" = cluster{"cycles":i32, "delay [s]":dbl, "enabled":bool, "overhead [s]":dbl, "tot smpls":i64, "sub-rec":i32, "overhead [%]":dbl, "emulated":bool}
  T50 = typedef "F8588A Low Pass Filter.ctl" = enum16{"Off", "100 kHz", "3 MHz"}
  T51 = typedef "F8588A Phase Lock.ctl" = enum16{"Off", "1 MHz", "10 MHz"}
  T52 = typedef "F8588A Coupling.ctl" = enum16{"AC, 1 MOhm", "AC, 10 MOhm", "DC, 1 MOhm", "DC, 10 MOhm", "DC, auto"}
  T53 = typedef "3458A Virtual Digitizer.lvlib/3458A Sampling Rate.ctl" = cluster{"freq mode":T4, "fs [Hz]":dbl, "fref [Hz]":dbl, "mul":dbl, "div":dbl}
  T54 = typedef "3458A Sample Rate Mode.ctl" = enum16{"fs or Ts", "fs*M/N"}
  T55 = typedef "DSDLL Virtual Digitizer.lvlib/DSDLL Session.ctl" = cluster{"dsdll":T56, "channels":i32, "device id":i32, "channel idns":string[], "proc setup":T58, "samples count":i32, "fs [Hz]":dbl}
  T56 = typedef "dsdll.lvlib/dsdll_instance.ctl" = cluster{"dsdll path":path, "dsdll handle":u8[], "output devices":T57[], "capture devices":T57[]}
  T57 = typedef "dsdll.lvlib/dsdll_device_record.ctl" = cluster{"guid":u8[], "name":string}
  T58 = typedef "DSDLL Virtual Digitizer.lvlib/DSDLL Process Config.ctl" = cluster{"packet size [smpl]":i32, "current timeout [s]":dbl, "blk2blk timeout [s]":dbl, "event time":timestamp, "data queue":refnum<queue>, "stop notifier":refnum<notifier>, "proc ref":refnum<vi>}
  T59 = typedef "ADC Type.ctl" = enum16{"niScope", "3458A", "DirectSound DLL", "Keysight DSO", "cDAQ ADC", "CMI ADS127L21", "dummy"}
  T60 = typedef "SimAdc Config.ctl" = cluster{"channels":T61[], "range [V]":dbl, "Ts step [s]":dbl, "time [s]":dbl, "fs [Hz]":dbl, "count":i64, "smpl offset":i64, "set count":i64, "bit res":i32}
  T61 = typedef "SimAdc Channel Cfg.ctl" = cluster{"harmonics":dbl[][], "btn clear":bool, "noise":dbl, "fundamental [Hz]":dbl}
  T62 = typedef "ADC On Close Action.ctl" = enum16{"Immediate reset", "Delayed reset"}
  T63 = typedef "MPX Session.ctl" = cluster{"Type":T64, "gen com ssn":T65, "delay before [s]":dbl, "delay post [s]":dbl, "sequence":string[], "enabled":bool, "ref timestamp [s]":dbl, "idn string":string, "dev niScope":refnum<k15>, "niScope idx":i32, "QPMX ssn":T69, "VISA mux ssn":T72}
  T64 = typedef "MPX Type.ctl" = enum16{"Dummy", "Generic - COM port", "Generic - niScope PFI", "Generic - VISA commands", "QPMX"}
  T65 = typedef "GCOMM Session.ctl" = cluster{"visa":refnum<visa-resource-name>, "primary":T66, "secondary":T66, "channels":T67[]}
  T66 = typedef "GCOMM Signal.ctl" = enum16{"None", "DTR", "RTS"}
  T67 = typedef "GCOMM Virtual Channel.ctl" = cluster{"Primary:":T68, "Secondary:":T68, "btn clr":bool, "btn up":bool, "btn down":bool, "Tag:":string}
  T68 = typedef "GCOMM Logic State.ctl" = enum16{"OFF", "ON"}
  T69 = typedef "QPMX Session.ctl" = cluster{"visa":refnum<visa-resource-name>, "switch mode":T70, "sequence":bool[][], "timing delays":u32[], "polarity":T71, "ss delay (s)":dbl, "internal timer (s)":dbl, "Last loaded sequence file":path, "startup delay (s)":dbl}
  T70 = typedef "QPMX switch mode.ctl" = enum16{"Switched by TWM", "Switched by external clock", "Switched by internal clock"}
  T71 = typedef "QPMX polarity.ctl" = enum16{"Positive", "Negative"}
  T72 = typedef "GVISA Mux Session.ctl" = cluster{"VISA":refnum<visa-resource-name>, "paths":T73[], "idn command":string, "serial cfg":T74}
  T73 = typedef "GVISA Mux Path Entry.ctl" = cluster{"Tag:":string, "Command:":string, "btn clr":bool, "btn up":bool, "btn down":bool}
  T74 = typedef "met_serial_setup.ctl" = cluster{"Baud rate":i32, "Data bits":i32, "Parity":i32, "Stop bits":i32, "Flow control":i32, "End Mode Read":enum16{"None", "Last Bit", "TermChar"}, "End Mode Write":enum16{"None", "Last Bit", "TermChar"}, "Term character":u8, "Term enable":bool}
  T75 = typedef "KeDSO session.ctl" = cluster{"VISA":refnum<visa-resource-name>, "channels":T76[], "bw limit [Hz]":dbl, "resolution":T77, "trig noise reject":enum16{"Normal", "High Sensitivity"}, "N":i64, "trigger config":T78, "fs [Hz]":dbl, "timeout stop":timestamp, "waiting for opc":bool, "fetch offset [smpl]":i64, "abs timestamp":timestamp, "ranges [V]":dbl[], "decimation":dbl, "ext ref":bool, "emulate aperture":bool, "model":T80}
  T76 = typedef "KeDSO Virtual Channel.ctl" = cluster{"Channel":i32, "Range [Vpk]":dbl, "btn clr":bool, "btn up":bool, "btn down":bool, "Offset [V]":dbl, "Coupling":enum16{"DC", "DC50", "AC", "LFR1"}, "bw limit enab":bool}
  T77 = typedef "KeDSO High Resolution Mode.ctl" = enum16{"Basic", "High-res AUTO", "Min. 9-bits", "Min. 10-bits", "Min. 11-bits", "Min. 12-bits", "Fixed 11-bits", "Fixed 12-bits", "Fixed 13-bits", "Fixed 14-bits", "Fixed 15-bits", "Fixed 16-bits"}
  T78 = typedef "KeDSO Trigger Setup.ctl" = cluster{"trigger source":T79, "trigger slope":enum16{"Negative", "Positive", "Either"}, "level [V]":dbl, "hysteresis [V]":dbl, "pre-trig [%]":i32}
  T79 = typedef "KeDSO Trigger Source.ctl" = enum16{"Immediate", "Level", "AUX"}
  T80 = typedef "Agilent 90000 Series.lvlib/DSO type.ctl" = enum16{"DSO91304", "DSO91204", "DSO90804", "DSO90604", "DSO90404", "DSO90254", "DSA91304", "DSA91204", "DSA90804", "DSA90604", "DSA90404", "DSA90254", "DSO9104", "DSO9254", "DSO9404", "MSO9104", "MSO9254", "MSO9404", "MSO9064", "DSO9064", "DSOX91604", "DSOX92004", "DSOX92504", "DSOX92804", "DSOX93204", "DSO93004", "DSO9024H", "DSO9054H", "DSO9104H", "DSO9204H", "DSOS054A", "DSOS104A", "DSOS204A", "DSOS254A", "DSOS404A", "DSOS604A", "DSOS804A", "MSOS054A", "MSOS104A", "MSOS204A", "MSOS254A", "MSOS404A", "MSOS604A", "MSOS804A", "DSAX96204Q", "DSOX96204Q", "DSAX95004Q", "DSOX95004Q", "DSAX93304Q", "DSOX93304Q", "DSAX92504Q", "DSOX92504Q", "DSAX92004Q", "DSOX92004Q"}
  T81 = typedef "cDAQ Session.ctl" = cluster{"mclk [Hz]":dbl, "ADC task":refnum<k21>, "mclk reference":string, "fs [Hz]":dbl, "queue adc cmd":refnum<queue>, "queue adc data":refnum<queue>, "adc proc ref":refnum<vi>, "channels":T82[], "last channels":T82[], "timeout":timestamp, "N":i32, "mclk mode":T83, "ext mclk source":tag}
  T82 = typedef "cDAQ Virtual Channel.ctl" = cluster{"Device":tag, "Channel id":i32, "btn clr":bool, "btn up":bool, "btn down":bool}
  T83 = typedef "cDAQ Master Clock Mode.ctl" = enum16{"Free running", "Export master clock", "Import master clock"}
  T84 = typedef "CMI ADS127L21 - Session.ctl" = cluster{"VISA":refnum<visa-resource-name>, "chn list":i32[], "record size":i32, "phys. channels":i32, "adc fifo size":i32, "channels":T85[], "ext refclk?":bool, "fs [Hz]":dbl, "ext refclk [Hz]":dbl, "meas refclk [Hz]":dbl, "EXTOUT mode":T89, "EXTOUT polarity":T90, "EXTOUT divisor":i32}
  T85 = typedef "CMI ADS127L21 - Record Channel.ctl" = cluster{"Range":T86, "Channel":i32, "Mode":T87, "Impedance":T88}
  T86 = typedef "CMI ADS127L21 - Input Range.ctl" = enum16{"±1.65V", "±2V"}
  T87 = typedef "CMI ADS127L21 - Input Mode.ctl" = enum16{"Normal", "Inverted", "GND"}
  T88 = typedef "CMI ADS127L21 - Input Impedance.ctl" = enum16{"1M", "1k5"}
  T89 = typedef "CMI ADS127L21 - EXTOUT Mode.ctl" = enum16{"ADCCLK", "REFCLK", "SMPLCLK", "FIRST"}
  T90 = typedef "CMI ADS127L21 - EXTOUT Polarity.ctl" = enum16{"NORM", "INV"}
  T91 = typedef "3458A Virtual Digitizer.lvlib/3458A Capabilities.ctl" = cluster{"max samples count":i64, "max fs [Hz]":ext, "min fs [Hz]":ext, "Ts step [s]":ext, "max Ts [s]":ext, "min Ts [s]":ext, "allows streaming?":bool, "streaming on?":bool, "has level trig?":bool, "has ext trig?":bool, "min aperture [s]":dbl, "max aperture [s]":dbl, "has aperture?":bool, "channels count":i32, "has temp.?":bool, "fs step [Hz]":ext, "const fs step?":bool, "no aper info":string, "has timestamps?":bool, "freq mode":T4, "auto aperture?":bool, "can select fs mode?":bool}
  T92 = typedef "niScope Virtual Digitizer.lvlib/niScope Capabilities.ctl" = cluster{"max samples count":i64, "max fs [Hz]":ext, "min fs [Hz]":ext, "Ts step [s]":ext, "max Ts [s]":ext, "min Ts [s]":ext, "allows streaming?":bool, "streaming on?":bool, "has level trig?":bool, "has ext trig?":bool, "channels count":i32, "has ranges?":bool}
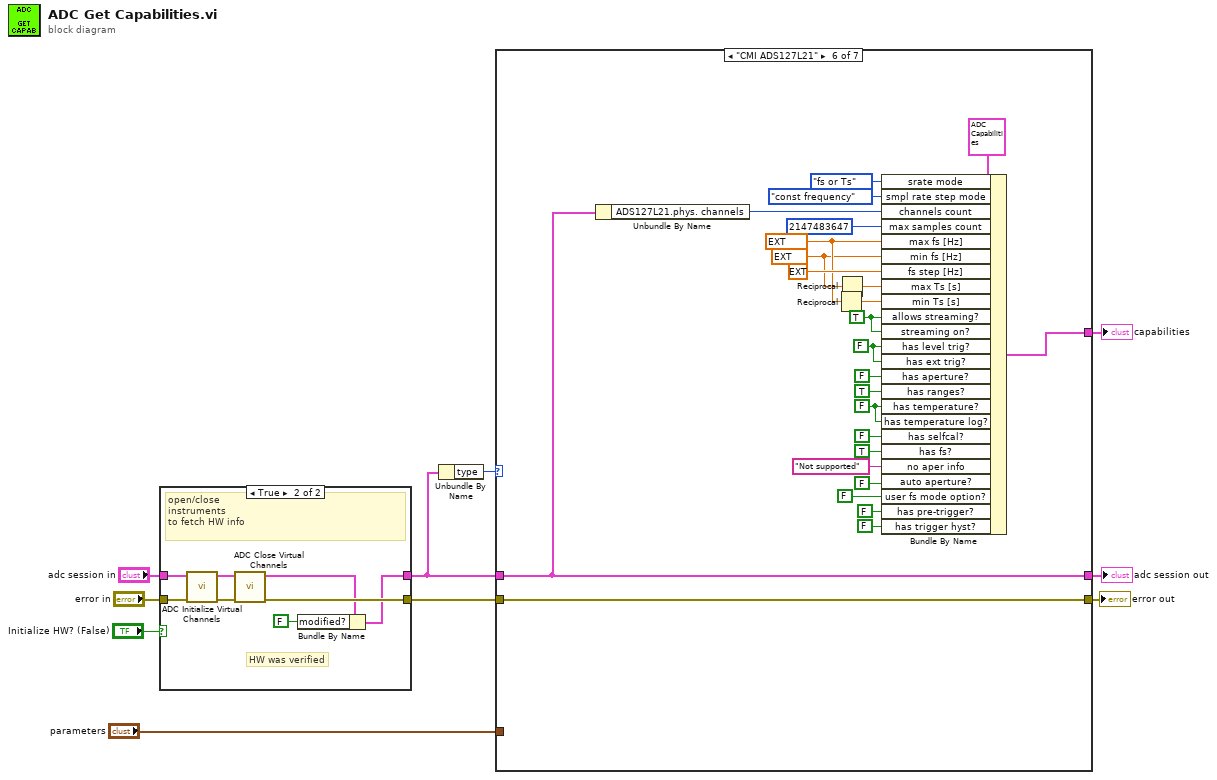
[diagram p0: block diagram]
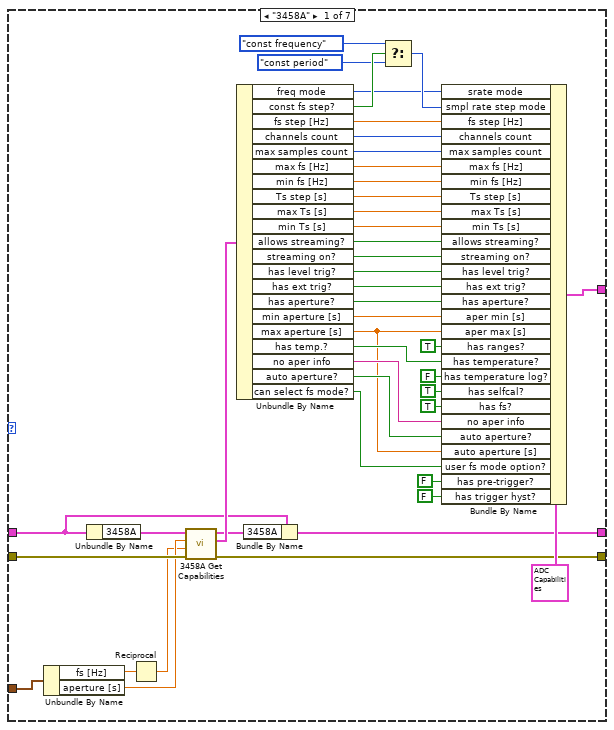
[diagram p2: hidden frame]
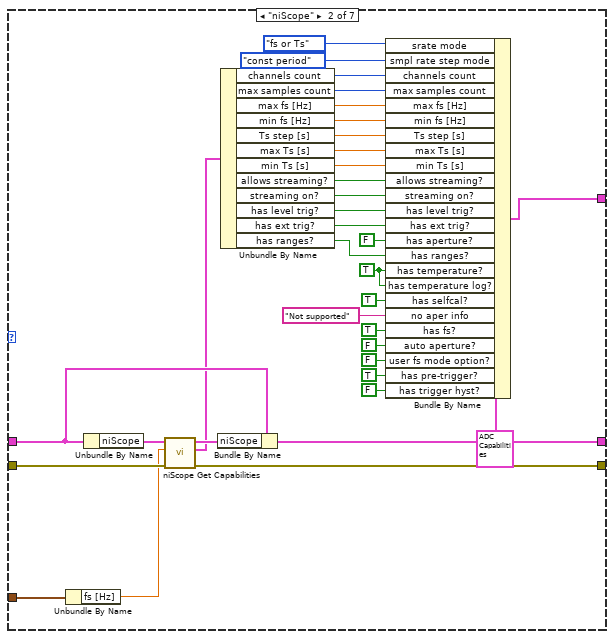
[diagram p3: hidden frame]
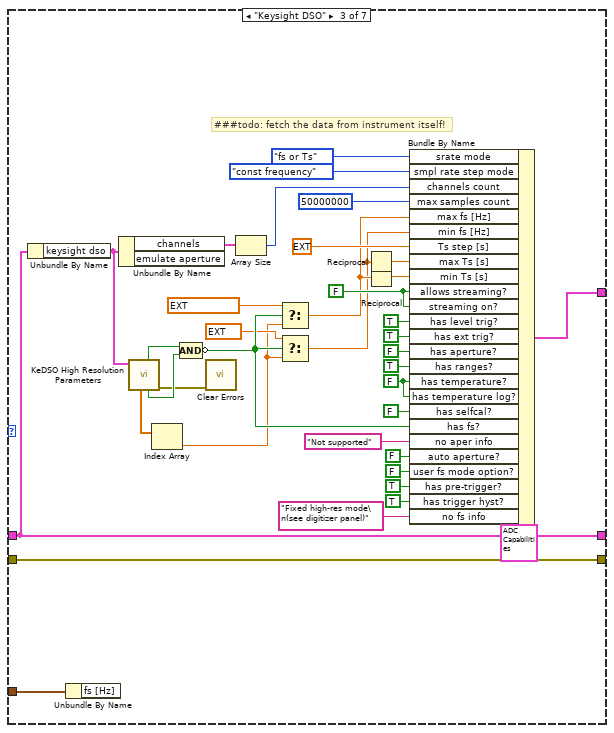
[diagram p4: hidden frame]
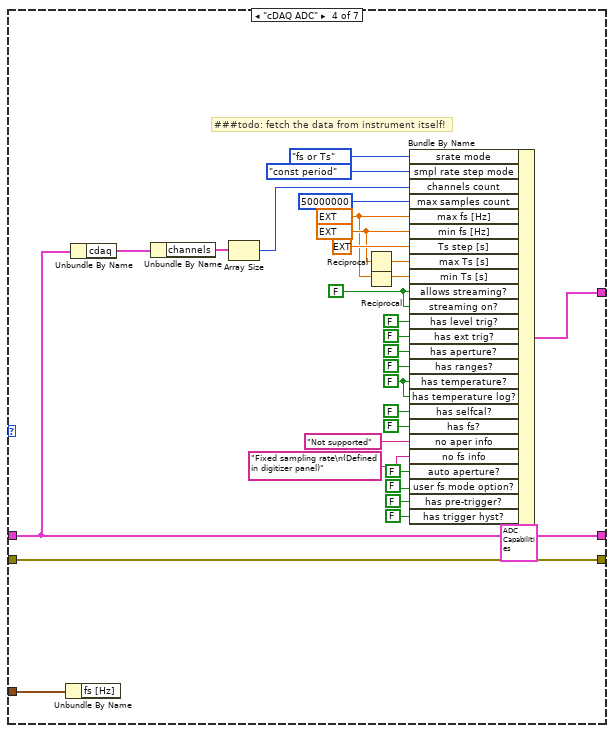
[diagram p5: hidden frame]
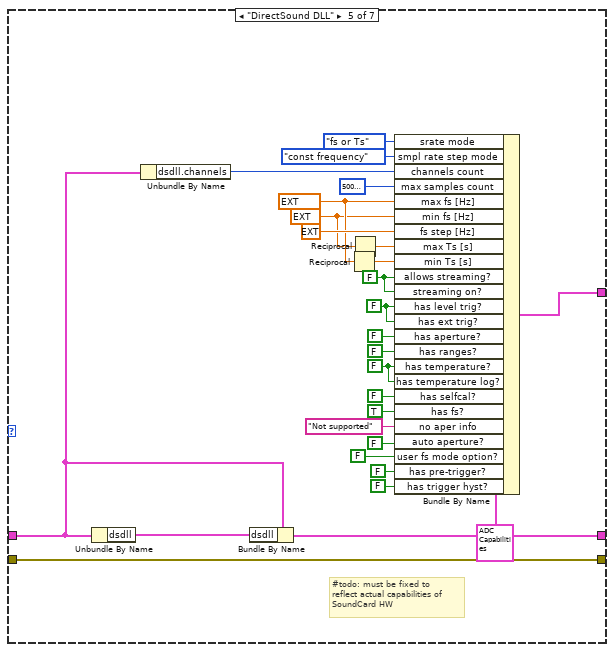
[diagram p6: hidden frame]
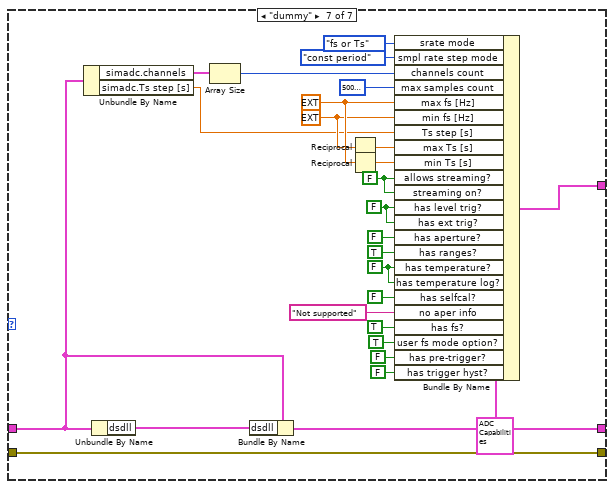
[diagram p7: hidden frame]
diagram:
  n1 = case shown="True" "Initialize HW? (False)" {
    tunnel: "error in" -> [w11 w20]
    tunnel: "adc session in" -> [w12 w17]
    tunnel: [w11 w16] -> w6
    tunnel: [w12 w15] -> w5
    frame False {
    }
    frame True {
      # "HW was verified"
      # "open/close\ninstruments\nto fetch HW info"
      n2 = call "ADC Initialize Virtual Channels.vi"("error in"=w20, "adc session in"=w17) -> ("error out"=w19:errorcluster, "adc session out"=w18:T5)  [unwired: 4 in, 4 out]
      n3 = call "ADC Close Virtual Channels.vi"("error in"=w19, "adc session in"=w18) -> ("error out"=w16:errorcluster, "adc session out"=w14:T5)  [unwired: 8 in]
      n4 = Bundle By Name(cluster=w14, "modified?"=FALSE) -> (w15:T5)
    }
  }
  n5 = Unbundle By Name(w5) -> ("type"=w7:T59)
  n6 = case shown="\"CMI ADS127L21\"" w7 {
    tunnel: w6 -> [w63 w83 w126 w156 w176 w204 w229]
    tunnel: w5 -> [w48 w85 w127 w157 w186 w192 w238]
    tunnel: [w49 w79 w126 w156 w176 w204 w229] -> w4
    tunnel: [w46 w84 w127 w157 w189 w192 w241] -> w3
    tunnel: [w45 w78 w132 w162 w188 w214 w240] -> w2
    tunnel: "parameters" -> [w44 w77 w131 w161 _ _ _]
    frame "3458A" {
      n7 = Unbundle By Name(w44) -> ("fs [Hz]"=w40:dbl, "aperture [s]"=w43:dbl)
      n8 = Unbundle By Name(w48) -> ("3458A"=w62:T17)
      n9 = Reciprocal(x=w40) -> (1/x=w39:dbl)
      n10 = call "3458A Get Capabilities.vi"("error in"=w63, "Ts [s]"=w39, "aperture [s]"=w43, "digitizer session in"=w62) -> ("error out"=w49:errorcluster, "capabilities"=w61:T91, "digitizer session out"=w47:T17)  [unwired: 5 in]
      n11 = Unbundle By Name(w61) -> ("freq mode"=w26:T4, "const fs step?"=w31:bool, "fs step [Hz]"=w33:ext, "channels count"=w38:i32, "max samples count"=w59:i64, "max fs [Hz]"=w58:ext, "min fs [Hz]"=w57:ext, "Ts step [s]"=w56:ext, "max Ts [s]"=w55:ext, "min Ts [s]"=w54:ext, "allows streaming?"=w53:bool, "streaming on?"=w52:bool, "has level trig?"=w51:bool, "has ext trig?"=w50:bool, "has aperture?"=w42:bool, "min aperture [s]"=w41:dbl, "max aperture [s]"=w24:dbl, "has temp.?"=w35:bool, "no aper info"=w27:string, "auto aperture?"=w25:bool, "can select fs mode?"=w23:bool)
      n12 = Bundle By Name(cluster=w48, "3458A"=w47) -> (w46:T5)
      n13 = Select(t=ADC_Sampling_Rate_Step_Mode."const frequency" ("smpl rate step mode"), s=w31, f=ADC_Sampling_Rate_Step_Mode."const period" ("smpl rate step mode")) -> (s? t:f=w32:T3)
      n14 = Bundle By Name(cluster=T2 {"max samples count"=0, "max fs [Hz]"=0.0, "min fs [Hz]"=0.0, "Ts step [s]"=0.0, "max Ts [s]"=0.0, "min Ts [s]"=0.0, "allows streaming?"=FALSE, "streaming on?"=FALSE, "has level trig?"=FALSE, "has ext trig?"=FALSE, "has aperture?"=FALSE, "aper min [s]"=0.0, "aper max [s]"=0.0, "channels count"=0, "has ranges?"=FALSE, "has temperature?"=FALSE, "has temperature log?"=FALSE, "has selfcal?"=FALSE, "fs step [Hz]"=0.0, "smpl rate step mode"=enum."const period", "no aper info"="", "no fs info"="", "has fs?"=FALSE, "srate mode"=enum."fs or Ts", "auto aperture?"=FALSE, "auto aperture [s]"=0.0, "user fs mode option?"=FALSE, "has pre-trigger?"=FALSE, "has trigger hyst?"=FALSE} ("capabilities"), "srate mode"=w26, "smpl rate step mode"=w32, "fs step [Hz]"=w33, "channels count"=w38, "max samples count"=w59, "max fs [Hz]"=w58, "min fs [Hz]"=w57, "Ts step [s]"=w56, "max Ts [s]"=w55, "min Ts [s]"=w54, "allows streaming?"=w53, "streaming on?"=w52, "has level trig?"=w51, "has ext trig?"=w50, "has aperture?"=w42, "aper min [s]"=w41, "aper max [s]"=w24, "has ranges?"=TRUE, "has temperature?"=w35, "has temperature log?"=FALSE, "has selfcal?"=TRUE, "has fs?"=TRUE, "no aper info"=w27, "auto aperture?"=w25, "auto aperture [s]"=w24, "user fs mode option?"=w23, "has pre-trigger?"=FALSE, "has trigger hyst?"=FALSE) -> (w45:T2)
    }
    frame "niScope" {
      w73 = TRUE ("has temperature?")
      n15 = Unbundle By Name(w77) -> ("fs [Hz]"=w76:dbl)
      n16 = Unbundle By Name(w85) -> ("niScope"=w82:T6)
      n17 = call "niScope Get Capabilities.vi"("error in"=w83, "fs [Hz]"=w76, "niScope session in"=w82) -> ("error out"=w79:errorcluster, "capabilities"=w80:T92, "niScope session out"=w81:T6)  [unwired: 6 in]
      n18 = Bundle By Name(cluster=w85, "niScope"=w81) -> (w84:T5)
      n19 = Unbundle By Name(w80) -> ("channels count"=w75:i32, "max samples count"=w96:i64, "max fs [Hz]"=w95:ext, "min fs [Hz]"=w94:ext, "Ts step [s]"=w93:ext, "max Ts [s]"=w92:ext, "min Ts [s]"=w91:ext, "allows streaming?"=w90:bool, "streaming on?"=w89:bool, "has level trig?"=w88:bool, "has ext trig?"=w87:bool, "has ranges?"=w74:bool)
      n20 = Bundle By Name(cluster=T2 {"max samples count"=0, "max fs [Hz]"=0.0, "min fs [Hz]"=0.0, "Ts step [s]"=0.0, "max Ts [s]"=0.0, "min Ts [s]"=0.0, "allows streaming?"=FALSE, "streaming on?"=FALSE, "has level trig?"=FALSE, "has ext trig?"=FALSE, "has aperture?"=FALSE, "aper min [s]"=0.0, "aper max [s]"=0.0, "channels count"=0, "has ranges?"=FALSE, "has temperature?"=FALSE, "has temperature log?"=FALSE, "has selfcal?"=FALSE, "fs step [Hz]"=0.0, "smpl rate step mode"=enum."const period", "no aper info"="", "no fs info"="", "has fs?"=FALSE, "srate mode"=enum."fs or Ts", "auto aperture?"=FALSE, "auto aperture [s]"=0.0, "user fs mode option?"=FALSE, "has pre-trigger?"=FALSE, "has trigger hyst?"=FALSE} ("capabilities"), "srate mode"=AWG_Clock_Setup_Mode."fs or Ts", "smpl rate step mode"=ADC_Sampling_Rate_Step_Mode."const period", "channels count"=w75, "max samples count"=w96, "max fs [Hz]"=w95, "min fs [Hz]"=w94, "Ts step [s]"=w93, "max Ts [s]"=w92, "min Ts [s]"=w91, "allows streaming?"=w90, "streaming on?"=w89, "has level trig?"=w88, "has ext trig?"=w87, "has aperture?"=FALSE, "has ranges?"=w74, "has temperature?"=w73, "has temperature log?"=w73, "has selfcal?"=TRUE, "no aper info"="Not supported", "has fs?"=TRUE, "auto aperture?"=FALSE, "user fs mode option?"=FALSE, "has pre-trigger?"=TRUE, "has trigger hyst?"=FALSE) -> (w78:T2)
    }
    frame "Keysight DSO" {
      w119 = FALSE ("allows streaming?")
      w130 = FALSE ("has temperature?")
      # "###todo: fetch the data from instrument itself!"
      n21 = Unbundle By Name(w127) -> ("keysight dso"=w109:T75)
      n22 = Unbundle By Name(w131) -> ()  [unwired: 1 out]
      n23 = Unbundle By Name(w109) -> ("channels"=w125:T76[])  [unwired: 1 out]
      n24 = call "KeDSO High Resolution Parameters.vi"("keysight dso"=w109) -> ("error out"=w99:errorcluster, "fixed bits?"=w106:bool, "fs info valid?"=w107:bool, "fs list [Hz]"=w108:dbl[])  [unwired: 4 in, 3 out]
      n25 = Index Array(array=w108) -> (element=w100:dbl)  [unwired: 1 in]
      n26 = Compound Arithmetic op=AND(w107, w106) -> (invert w104:bool)
      n27 = call <vilib>:"Clear Errors.vi"("error in (no error)"=w99) -> ()  [unwired: 5 in, 2 out]
      n28 = Array Size(array=w125) -> (size(s)=w124:i32)
      n29 = Select(t=ext 20000000000.0 ("max fs [Hz]"), s=w104, f=w100) -> (s? t:f=w102:ext)
      n30 = Select(t=ext 50000.0 ("min fs [Hz]"), s=w104, f=w100) -> (s? t:f=w101:ext)
      n31 = Reciprocal(x=w101) -> (1/x=w121:ext)
      n32 = Reciprocal(x=w102) -> (1/x=w120:ext)
      n33 = Bundle By Name(cluster=T2 {"max samples count"=0, "max fs [Hz]"=0.0, "min fs [Hz]"=0.0, "Ts step [s]"=0.0, "max Ts [s]"=0.0, "min Ts [s]"=0.0, "allows streaming?"=FALSE, "streaming on?"=FALSE, "has level trig?"=FALSE, "has ext trig?"=FALSE, "has aperture?"=FALSE, "aper min [s]"=0.0, "aper max [s]"=0.0, "channels count"=0, "has ranges?"=FALSE, "has temperature?"=FALSE, "has temperature log?"=FALSE, "has selfcal?"=FALSE, "fs step [Hz]"=0.0, "smpl rate step mode"=enum."const period", "no aper info"="", "no fs info"="", "has fs?"=FALSE, "srate mode"=enum."fs or Ts", "auto aperture?"=FALSE, "auto aperture [s]"=0.0, "user fs mode option?"=FALSE, "has pre-trigger?"=FALSE, "has trigger hyst?"=FALSE} ("capabilities"), "srate mode"=AWG_Clock_Setup_Mode."fs or Ts", "smpl rate step mode"=ADC_Sampling_Rate_Step_Mode."const frequency", "channels count"=w124, "max samples count"=i64 50000000, "max fs [Hz]"=w102, "min fs [Hz]"=w101, "Ts step [s]"=ext 1.0, "max Ts [s]"=w121, "min Ts [s]"=w120, "allows streaming?"=w119, "streaming on?"=w119, "has level trig?"=TRUE, "has ext trig?"=TRUE, "has aperture?"=FALSE, "has ranges?"=TRUE, "has temperature?"=w130, "has temperature log?"=w130, "has selfcal?"=FALSE, "has fs?"=w104, "no aper info"="Not supported", "auto aperture?"=FALSE, "user fs mode option?"=FALSE, "has pre-trigger?"=TRUE, "has trigger hyst?"=TRUE, "no fs info"="Fixed high-res mode\n(see digitizer panel)") -> (w132:T2)
    }
    frame "cDAQ ADC" {
      w146 = FALSE ("allows streaming?")
      w150 = ext 50000.0 ("min fs [Hz]")
      w147 = ext 50000.0 ("max fs [Hz]")
      w160 = FALSE ("has temperature?")
      # "###todo: fetch the data from instrument itself!"
      n34 = Unbundle By Name(w161) -> ()  [unwired: 1 out]
      n35 = Unbundle By Name(w157) -> ("cdaq"=w155:T81)
      n36 = Unbundle By Name(w155) -> ("channels"=w154:T82[])
      n37 = Array Size(array=w154) -> (size(s)=w153:i32)
      n38 = Reciprocal(x=w150) -> (1/x=w149:ext)
      n39 = Reciprocal(x=w147) -> (1/x=w148:ext)
      n40 = Bundle By Name(cluster=T2 {"max samples count"=0, "max fs [Hz]"=0.0, "min fs [Hz]"=0.0, "Ts step [s]"=0.0, "max Ts [s]"=0.0, "min Ts [s]"=0.0, "allows streaming?"=FALSE, "streaming on?"=FALSE, "has level trig?"=FALSE, "has ext trig?"=FALSE, "has aperture?"=FALSE, "aper min [s]"=0.0, "aper max [s]"=0.0, "channels count"=0, "has ranges?"=FALSE, "has temperature?"=FALSE, "has temperature log?"=FALSE, "has selfcal?"=FALSE, "fs step [Hz]"=0.0, "smpl rate step mode"=enum."const period", "no aper info"="", "no fs info"="", "has fs?"=FALSE, "srate mode"=enum."fs or Ts", "auto aperture?"=FALSE, "auto aperture [s]"=0.0, "user fs mode option?"=FALSE, "has pre-trigger?"=FALSE, "has trigger hyst?"=FALSE} ("capabilities"), "srate mode"=AWG_Clock_Setup_Mode."fs or Ts", "smpl rate step mode"=ADC_Sampling_Rate_Step_Mode."const period", "channels count"=w153, "max samples count"=i64 50000000, "max fs [Hz]"=w147, "min fs [Hz]"=w150, "Ts step [s]"=ext 1.0, "max Ts [s]"=w149, "min Ts [s]"=w148, "allows streaming?"=w146, "streaming on?"=w146, "has level trig?"=FALSE, "has ext trig?"=FALSE, "has aperture?"=FALSE, "has ranges?"=FALSE, "has temperature?"=w160, "has temperature log?"=w160, "has selfcal?"=FALSE, "has fs?"=FALSE, "no aper info"="Not supported", "no fs info"="Fixed sampling rate\n(Defined in digitizer panel)", "auto aperture?"=FALSE, "user fs mode option?"=FALSE, "has pre-trigger?"=FALSE, "has trigger hyst?"=FALSE) -> (w162:T2)
    }
    frame "DirectSound DLL" {
      w174 = FALSE ("has temperature?")
      w177 = FALSE ("has level trig?")
      w178 = FALSE ("allows streaming?")
      w179 = ext 8000.0 ("min fs [Hz]")
      w182 = ext 192000.0 ("max fs [Hz]")
      # "#todo: must be fixed to \nreflect actual capabilities of\nSoundCard HW"
      n41 = Unbundle By Name(w186) -> ("dsdll"=w187:T55)
      n42 = Unbundle By Name(w186) -> ("dsdll.channels"=w185:i32)
      n43 = Bundle By Name(cluster=w186, "dsdll"=w187) -> (w189:T5)
      n44 = Reciprocal(x=w182) -> (1/x=w181:ext)
      n45 = Reciprocal(x=w179) -> (1/x=w180:ext)
      n46 = Bundle By Name(cluster=T2 {"max samples count"=0, "max fs [Hz]"=0.0, "min fs [Hz]"=0.0, "Ts step [s]"=0.0, "max Ts [s]"=0.0, "min Ts [s]"=0.0, "allows streaming?"=FALSE, "streaming on?"=FALSE, "has level trig?"=FALSE, "has ext trig?"=FALSE, "has aperture?"=FALSE, "aper min [s]"=0.0, "aper max [s]"=0.0, "channels count"=0, "has ranges?"=FALSE, "has temperature?"=FALSE, "has temperature log?"=FALSE, "has selfcal?"=FALSE, "fs step [Hz]"=0.0, "smpl rate step mode"=enum."const period", "no aper info"="", "no fs info"="", "has fs?"=FALSE, "srate mode"=enum."fs or Ts", "auto aperture?"=FALSE, "auto aperture [s]"=0.0, "user fs mode option?"=FALSE, "has pre-trigger?"=FALSE, "has trigger hyst?"=FALSE} ("capabilities"), "srate mode"=AWG_Clock_Setup_Mode."fs or Ts", "smpl rate step mode"=ADC_Sampling_Rate_Step_Mode."const frequency", "channels count"=w185, "max samples count"=50000000, "max fs [Hz]"=w182, "min fs [Hz]"=w179, "fs step [Hz]"=ext 1.0 ("Ts step [s]"), "max Ts [s]"=w180, "min Ts [s]"=w181, "allows streaming?"=w178, "streaming on?"=w178, "has level trig?"=w177, "has ext trig?"=w177, "has aperture?"=FALSE, "has ranges?"=FALSE, "has temperature?"=w174, "has temperature log?"=w174, "has selfcal?"=FALSE, "has fs?"=TRUE, "no aper info"="Not supported", "auto aperture?"=FALSE, "user fs mode option?"=FALSE, "has pre-trigger?"=FALSE, "has trigger hyst?"=FALSE) -> (w188:T2)
    }
    frame "CMI ADS127L21" {
      w202 = FALSE ("has temperature?")
      w205 = FALSE ("has level trig?")
      w206 = TRUE ("allows streaming?")
      w207 = ext 50000.0 ("min fs [Hz]")
      w210 = ext 406250.0 ("max fs [Hz]")
      n47 = Unbundle By Name(w192) -> ("ADS127L21.phys. channels"=w213:i32)
      n48 = Reciprocal(x=w210) -> (1/x=w209:ext)
      n49 = Reciprocal(x=w207) -> (1/x=w208:ext)
      n50 = Bundle By Name(cluster=T2 {"max samples count"=0, "max fs [Hz]"=0.0, "min fs [Hz]"=0.0, "Ts step [s]"=0.0, "max Ts [s]"=0.0, "min Ts [s]"=0.0, "allows streaming?"=FALSE, "streaming on?"=FALSE, "has level trig?"=FALSE, "has ext trig?"=FALSE, "has aperture?"=FALSE, "aper min [s]"=0.0, "aper max [s]"=0.0, "channels count"=0, "has ranges?"=FALSE, "has temperature?"=FALSE, "has temperature log?"=FALSE, "has selfcal?"=FALSE, "fs step [Hz]"=0.0, "smpl rate step mode"=enum."const period", "no aper info"="", "no fs info"="", "has fs?"=FALSE, "srate mode"=enum."fs or Ts", "auto aperture?"=FALSE, "auto aperture [s]"=0.0, "user fs mode option?"=FALSE, "has pre-trigger?"=FALSE, "has trigger hyst?"=FALSE} ("capabilities"), "srate mode"=AWG_Clock_Setup_Mode."fs or Ts", "smpl rate step mode"=ADC_Sampling_Rate_Step_Mode."const frequency", "channels count"=w213, "max samples count"=2147483647, "max fs [Hz]"=w210, "min fs [Hz]"=w207, "fs step [Hz]"=ext 1.0 ("Ts step [s]"), "max Ts [s]"=w208, "min Ts [s]"=w209, "allows streaming?"=w206, "streaming on?"=w206, "has level trig?"=w205, "has ext trig?"=w205, "has aperture?"=FALSE, "has ranges?"=TRUE, "has temperature?"=w202, "has temperature log?"=w202, "has selfcal?"=FALSE, "has fs?"=TRUE, "no aper info"="Not supported", "auto aperture?"=FALSE, "user fs mode option?"=FALSE, "has pre-trigger?"=FALSE, "has trigger hyst?"=FALSE) -> (w214:T2)
    }
    frame "dummy" {
      w227 = FALSE ("has temperature?")
      w230 = FALSE ("has level trig?")
      w231 = FALSE ("allows streaming?")
      w232 = ext 1.0 ("min fs [Hz]")
      w235 = ext 1000000000.0 ("max fs [Hz]")
      n51 = Unbundle By Name(w238) -> ("simadc.channels"=w237:T61[], "simadc.Ts step [s]"=w224:dbl)
      n52 = Unbundle By Name(w238) -> ("dsdll"=w239:T55)
      n53 = Array Size(array=w237) -> (size(s)=w225:i32)
      n54 = Bundle By Name(cluster=w238, "dsdll"=w239) -> (w241:T5)
      n55 = Reciprocal(x=w232) -> (1/x=w233:ext)
      n56 = Reciprocal(x=w235) -> (1/x=w234:ext)
      n57 = Bundle By Name(cluster=T2 {"max samples count"=0, "max fs [Hz]"=0.0, "min fs [Hz]"=0.0, "Ts step [s]"=0.0, "max Ts [s]"=0.0, "min Ts [s]"=0.0, "allows streaming?"=FALSE, "streaming on?"=FALSE, "has level trig?"=FALSE, "has ext trig?"=FALSE, "has aperture?"=FALSE, "aper min [s]"=0.0, "aper max [s]"=0.0, "channels count"=0, "has ranges?"=FALSE, "has temperature?"=FALSE, "has temperature log?"=FALSE, "has selfcal?"=FALSE, "fs step [Hz]"=0.0, "smpl rate step mode"=enum."const period", "no aper info"="", "no fs info"="", "has fs?"=FALSE, "srate mode"=enum."fs or Ts", "auto aperture?"=FALSE, "auto aperture [s]"=0.0, "user fs mode option?"=FALSE, "has pre-trigger?"=FALSE, "has trigger hyst?"=FALSE} ("capabilities"), "srate mode"=AWG_Clock_Setup_Mode."fs or Ts", "smpl rate step mode"=ADC_Sampling_Rate_Step_Mode."const period", "channels count"=w225, "max samples count"=50000000, "max fs [Hz]"=w235, "min fs [Hz]"=w232, "Ts step [s]"=w224, "max Ts [s]"=w233, "min Ts [s]"=w234, "allows streaming?"=w231, "streaming on?"=w231, "has level trig?"=w230, "has ext trig?"=w230, "has aperture?"=FALSE, "has ranges?"=TRUE, "has temperature?"=w227, "has temperature log?"=w227, "has selfcal?"=FALSE, "no aper info"="Not supported", "has fs?"=TRUE, "user fs mode option?"=TRUE, "has pre-trigger?"=FALSE, "has trigger hyst?"=FALSE) -> (w240:T2)
    }
  }
  "error out" <- w4
  "adc session out" <- w3
  "capabilities" <- w2
